vi "QPD Image Plane.vi"() -> ()   [LabVIEW 2018]
panel:
  in  "stop":bool
  out "Beam Centering 2":cluster{"Y":dbl[], "Y":dbl[]}[](graph) caption="Beam Centering"
  out "RF Offset A":dbl format="%0.6f"
  out "RF Offset C":dbl format="%0.6f"
  out "RF Offset B":dbl format="%0.6f"
  out "RF Offset D":dbl format="%0.6f"
  out "A":dynamicdata(graph)
  out "DC Offset A":dbl format="%0.6f"
  out "DC Offset C":dbl format="%0.6f"
  out "DC Offset B":dbl format="%0.6f"
  out "DC Offset D":dbl format="%0.6f"
  out "DC Responsivity D":dbl
  out "DC Responsivity C":dbl
  out "DC Responsivity B":dbl
  out "DC Responsivity A":dbl
  out "DC Responsivity D":dbl
  out "DC Responsivity C":dbl
  out "DC Responsivity B":dbl
  out "DC Responsivity A":dbl
  out "Y: (A+C)-(B+D)":dynamicdata(graph)
  out "X: (A+B)-(C+D)":dynamicdata(graph)
  out "D":dynamicdata(graph)
  out "B":dynamicdata(graph)
  out "C":dynamicdata(graph)
  out "Beam Centering":cluster{"Y":dbl[], "Y":dbl[]}[](graph)
  out "Y: (A+C)-(B+D)":dynamicdata(graph)
  out "X: (A+B)-(C+D)":dynamicdata(graph)
  out "Saving Data":bool
  out "Filename Out":path
  in  "Filename":path=path "C:/Users/physics-svc-fulda/Desktop/Data.lvm"
  in  "Enable":bool=TRUE
  out "D":dynamicdata(graph)
  out "B":dynamicdata(graph)
  out "C":dynamicdata(graph)
  out "A":dynamicdata(graph)
  in  "timeout (s)":dbl=10.0 format="%0.2f"
  in  "rate":dbl=1000.0
  in  "# of samples":i32=100
  out "Combined":dynamicdata(graph)
  # "Rayleigh Length"
  # "PZT Image Plane"
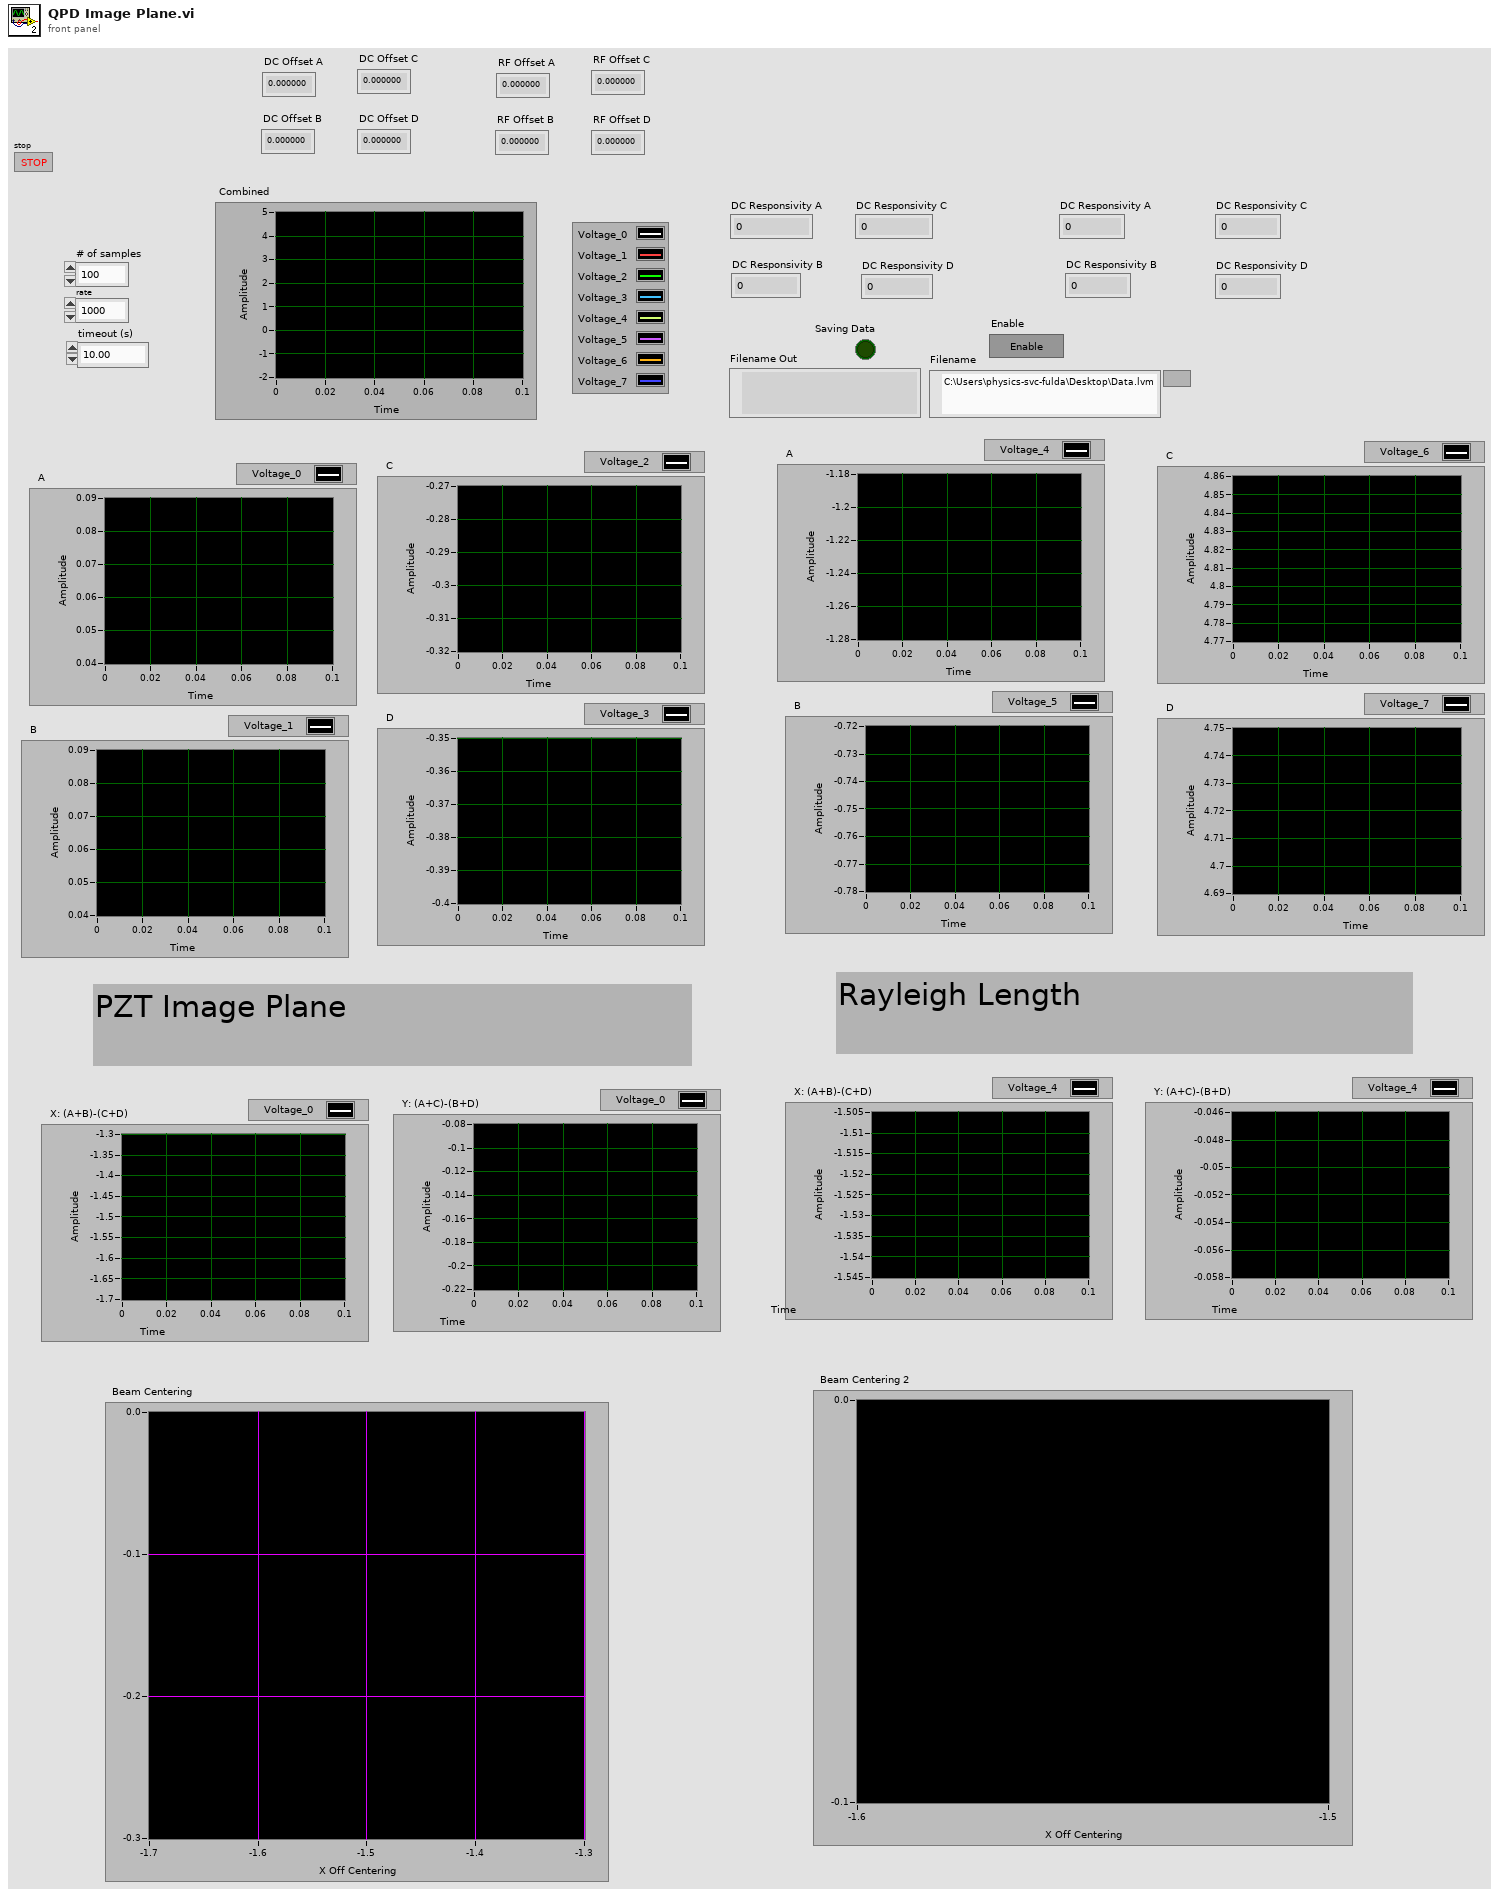
[diagram p1: front panel]
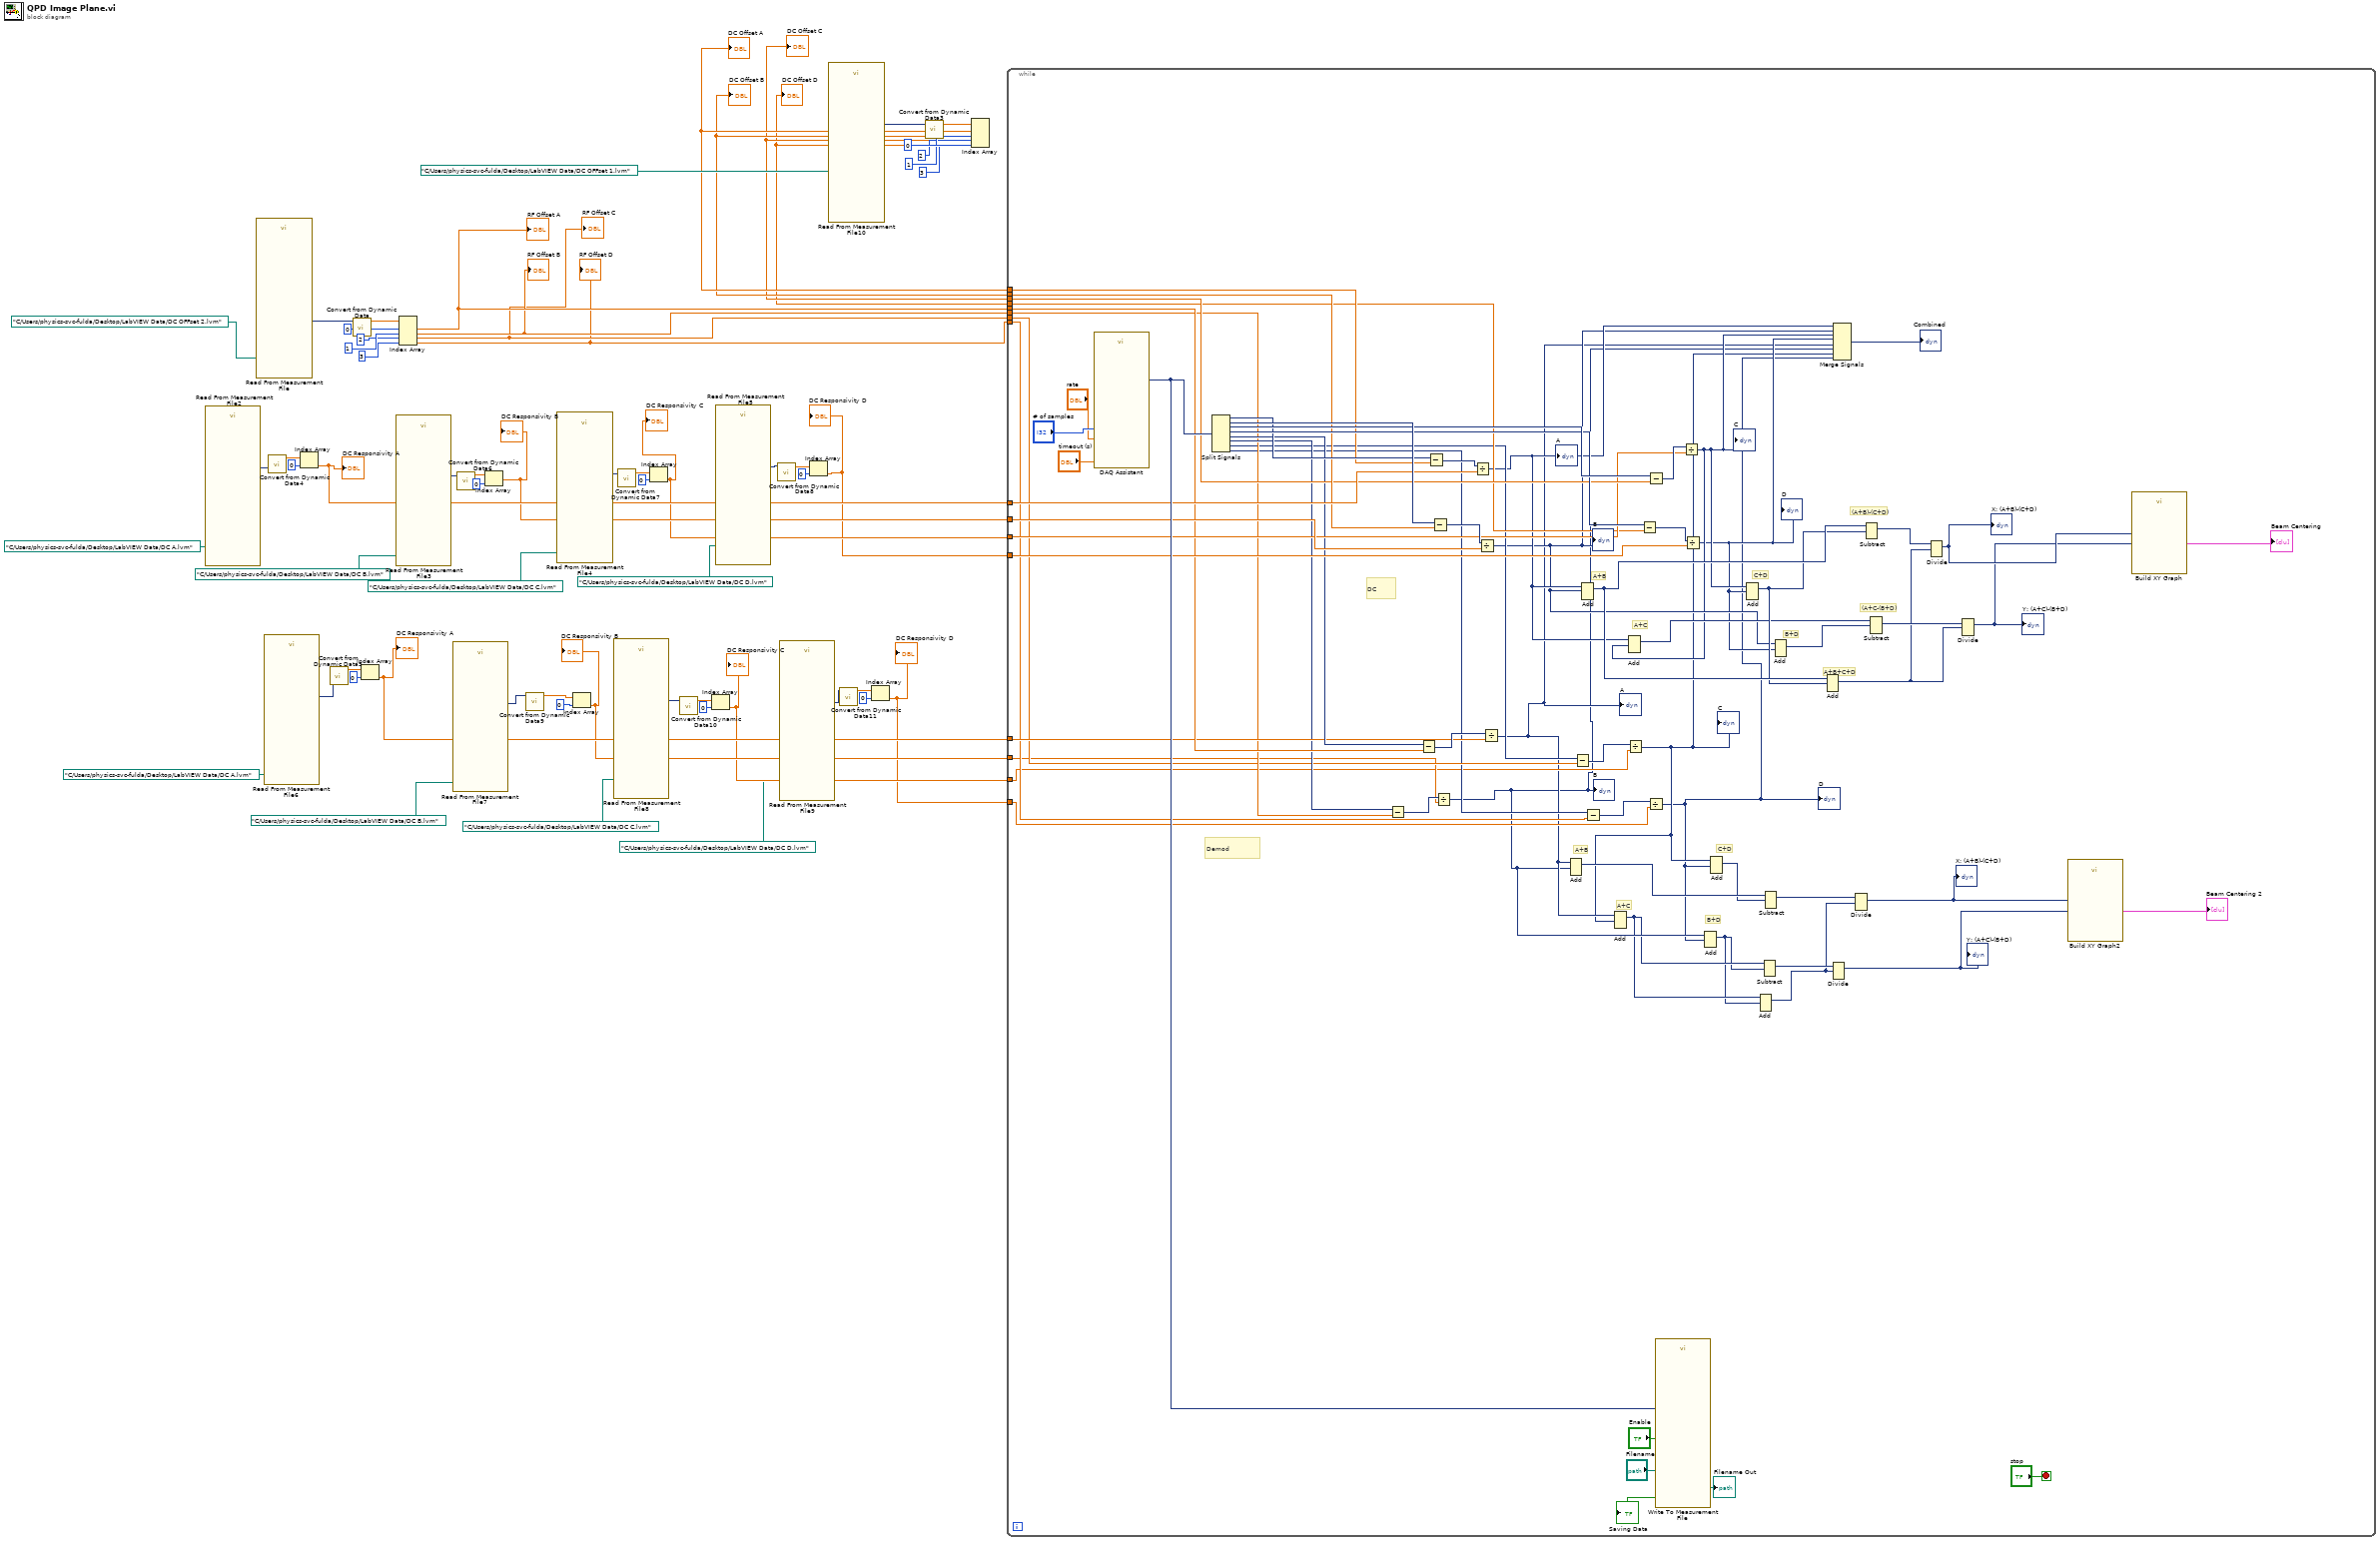
[diagram p0: block diagram]
diagram:
  n1 = call "Read From Measurement File2"("Filename"=path "C:/Users/physics-svc-fulda/Desktop/LabVIEW Data/DC A.lvm") -> ("Signals"=w46:dynamicdata)  [unwired: 5 in, 5 out]
  n2 = call "Read From Measurement File"("Filename"=path "C:/Users/physics-svc-fulda/Desktop/LabVIEW Data/DC OFFset 2.lvm") -> ("Signals"=w10:dynamicdata)  [unwired: 5 in, 5 out]
  n3 = call "Read From Measurement File6"("Filename"=path "C:/Users/physics-svc-fulda/Desktop/LabVIEW Data/DC A.lvm") -> ("Signals"=w49:dynamicdata)  [unwired: 5 in, 5 out]
  n4 = call "Convert from Dynamic Data4"("Dynamic Data Type"=w46) -> ("Array"=w47:dbl[])  [unwired: 3 in]
  n5 = Index Array(array=w47, index=0) -> (element=w31:dbl)
  "DC Responsivity A" <- w31
  n6 = call "Convert from Dynamic Data5"("Dynamic Data Type"=w49) -> ("Array"=w48:dbl[])  [unwired: 3 in]
  n7 = call "Convert from Dynamic Data"("Dynamic Data Type"=w10) -> ("Array"=w11:dbl[])  [unwired: 3 in]
  n8 = Index Array(array=w48, index=0) -> (element=w27:dbl)
  "DC Responsivity A" <- w27
  n9 = call "Read From Measurement File3"("Filename"=path "C:/Users/physics-svc-fulda/Desktop/LabVIEW Data/DC B.lvm") -> ("Signals"=w51:dynamicdata)  [unwired: 5 in, 5 out]
  n10 = Index Array(array=w11, index #1=0 ("index"), index #2=1 ("index"), index #3=2 ("index"), index #4=3 ("index")) -> (element #1=w4:dbl, element #2=w3:dbl, element #3=w2:dbl, element #4=w1:dbl)
  "RF Offset D" <- w1
  "RF Offset B" <- w3
  "RF Offset C" <- w2
  "RF Offset A" <- w4
  n11 = call "Read From Measurement File7"("Filename"=path "C:/Users/physics-svc-fulda/Desktop/LabVIEW Data/DC B.lvm") -> ("Signals"=w38:dynamicdata)  [unwired: 5 in, 5 out]
  n12 = call "Convert from Dynamic Data6"("Dynamic Data Type"=w51) -> ("Array"=w50:dbl[])  [unwired: 3 in]
  n13 = Index Array(array=w50, index=0) -> (element=w30:dbl)
  "DC Responsivity B" <- w30
  n14 = call "Convert from Dynamic Data9"("Dynamic Data Type"=w38) -> ("Array"=w40:dbl[])  [unwired: 3 in]
  n15 = call "Read From Measurement File4"("Filename"=path "C:/Users/physics-svc-fulda/Desktop/LabVIEW Data/DC C.lvm") -> ("Signals"=w53:dynamicdata)  [unwired: 5 in, 5 out]
  n16 = Index Array(array=w40, index=0) -> (element=w26:dbl)
  "DC Responsivity B" <- w26
  n17 = call "Read From Measurement File8"("Filename"=path "C:/Users/physics-svc-fulda/Desktop/LabVIEW Data/DC C.lvm") -> ("Signals"=w33:dynamicdata)  [unwired: 5 in, 5 out]
  n18 = call "Convert from Dynamic Data7"("Dynamic Data Type"=w53) -> ("Array"=w52:dbl[])  [unwired: 3 in]
  n19 = Index Array(array=w52, index=0) -> (element=w29:dbl)
  "DC Responsivity C" <- w29
  n20 = call "Convert from Dynamic Data10"("Dynamic Data Type"=w33) -> ("Array"=w37:dbl[])  [unwired: 3 in]
  n21 = Index Array(array=w37, index=0) -> (element=w25:dbl)
  "DC Responsivity C" <- w25
  n22 = call "Read From Measurement File5"("Filename"=path "C:/Users/physics-svc-fulda/Desktop/LabVIEW Data/DC D.lvm") -> ("Signals"=w55:dynamicdata)  [unwired: 5 in, 5 out]
  n23 = call "Convert from Dynamic Data8"("Dynamic Data Type"=w55) -> ("Array"=w54:dbl[])  [unwired: 3 in]
  n24 = call "Read From Measurement File9"("Filename"=path "C:/Users/physics-svc-fulda/Desktop/LabVIEW Data/DC D.lvm") -> ("Signals"=w32:dynamicdata)  [unwired: 5 in, 5 out]
  n25 = Index Array(array=w54, index=0) -> (element=w28:dbl)
  "DC Responsivity D" <- w28
  n26 = call "Read From Measurement File10"("Filename"=path "C:/Users/physics-svc-fulda/Desktop/LabVIEW Data/DC OFFset 1.lvm") -> ("Signals"=w61:dynamicdata)  [unwired: 5 in, 5 out]
  n27 = call "Convert from Dynamic Data11"("Dynamic Data Type"=w32) -> ("Array"=w35:dbl[])  [unwired: 3 in]
  n28 = Index Array(array=w35, index=0) -> (element=w24:dbl)
  "DC Responsivity D" <- w24
  n29 = call "Convert from Dynamic Data3"("Dynamic Data Type"=w61) -> ("Array"=w62:dbl[])  [unwired: 3 in]
  n30 = Index Array(array=w62, index #1=0 ("index"), index #2=1 ("index"), index #3=2 ("index"), index #4=3 ("index")) -> (element #1=w23:dbl, element #2=w22:dbl, element #3=w21:dbl, element #4=w20:dbl)
  "DC Offset D" <- w20
  "DC Offset B" <- w22
  "DC Offset C" <- w21
  "DC Offset A" <- w23
  n31 = while {
    tunnel: w23 -> [w106]
    tunnel: w22 -> [w104]
    tunnel: w21 -> [w102]
    tunnel: w20 -> [w100]
    tunnel: w4 -> [w97]
    tunnel: w3 -> [w92]
    tunnel: w2 -> [w89]
    tunnel: w1 -> [w86]
    tunnel: w31 -> [w105]
    tunnel: w30 -> [w103]
    tunnel: w29 -> [w101]
    tunnel: w28 -> [w99]
    tunnel: w27 -> [w95]
    tunnel: w26 -> [w85]
    tunnel: w25 -> [w84]
    tunnel: w24 -> [w83]
    stop <- "stop" stop-if-true
    # "B+D"
    # "A+C"
    # "C+D"
    # "A+B"
    # "(A+C-(B+D)"
    # "(A+B)-(C+D)"
    # "A+B+C+D"
    # "B+D"
    # "A+C"
    # "C+D"
    # "A+B"
    # "Demod"
    # "DC"
    n32 = call "DAQ Assistant"("rate"="rate", "number of samples"="# of samples", "timeout (s)"="timeout (s)") -> ("data"=w125:dynamicdata)  [unwired: 14 in, 2 out]
    n33 = Split Signals(w125) -> (w108:dynamicdata, w123:dynamicdata, w121:dynamicdata, w119:dynamicdata, w98:dynamicdata, w93:dynamicdata, w90:dynamicdata, w87:dynamicdata)  [unwired: 8 in]
    n34 = Subtract(x=w93, y=w92) -> (x-y=w94:dynamicdata)
    n35 = Subtract(x=w98, y=w97) -> (x-y=w96:dynamicdata)
    n36 = Subtract(x=w108, y=w106) -> (x-y=w107:dynamicdata)
    n37 = Subtract(x=w123, y=w104) -> (x-y=w122:dynamicdata)
    n38 = Divide(x=w94, y=w85) -> (x/y=w74:dynamicdata)
    "B" <- w74
    n39 = Divide(x=w107, y=w105) -> (x/y=w79:dynamicdata)
    "A" <- w79
    n40 = Divide(x=w122, y=w103) -> (x/y=w78:dynamicdata)
    "B" <- w78
    n41 = Divide(x=w96, y=w95) -> (x/y=w75:dynamicdata)
    "A" <- w75
    n42 = Add(1:w74, 2:w75) -> (0:w82:dynamicdata)  [unwired: 1 in, 1 out]
    n43 = Subtract(x=w90, y=w89) -> (x-y=w91:dynamicdata)
    n44 = Add(1:w78, 2:w79) -> (0:w117:dynamicdata)  [unwired: 1 in, 1 out]
    n45 = Subtract(x=w87, y=w86) -> (x-y=w88:dynamicdata)
    n46 = Divide(x=w91, y=w84) -> (x/y=w73:dynamicdata)
    "C" <- w73
    n47 = Add(1:w73, 2:w75) -> (0:w71:dynamicdata)  [unwired: 1 in, 1 out]
    n48 = Subtract(x=w119, y=w100) -> (x-y=w118:dynamicdata)
    n49 = Divide(x=w88, y=w83) -> (x/y=w72:dynamicdata)
    "D" <- w72
    n50 = Subtract(x=w121, y=w102) -> (x-y=w120:dynamicdata)
    n51 = call "Write To Measurement File"("Signals"=w125, "Enable"="Enable", "Filename"="Filename") -> ("Filename Out"=→"Filename Out":path, "Saving Data"=→"Saving Data":bool)  [unwired: 14 in, 1 out]
    n52 = Divide(x=w120, y=w101) -> (x/y=w77:dynamicdata)
    "C" <- w77
    n53 = Add(1:w77, 2:w79) -> (0:w114:dynamicdata)  [unwired: 1 in, 1 out]
    n54 = Divide(x=w118, y=w99) -> (x/y=w76:dynamicdata)
    "D" <- w76
    n55 = Add(1:w72, 2:w74) -> (0:w70:dynamicdata)  [unwired: 1 in, 1 out]
    n56 = Add(1:w72, 2:w73) -> (0:w81:dynamicdata)  [unwired: 1 in, 1 out]
    n57 = Add(1:w76, 2:w77) -> (0:w116:dynamicdata)  [unwired: 1 in, 1 out]
    n58 = Add(1:w70, 2:w71) -> (0:w67:dynamicdata)  [unwired: 1 in, 1 out]
    n59 = Subtract(1:w70, 2:w71) -> (0:w68:dynamicdata)  [unwired: 1 in, 1 out]
    n60 = Subtract(1:w81, 2:w82) -> (0:w69:dynamicdata)  [unwired: 1 in, 1 out]
    n61 = Add(1:w76, 2:w78) -> (0:w113:dynamicdata)  [unwired: 1 in, 1 out]
    n62 = Add(1:w116, 2:w117) -> (0:w111:dynamicdata)  [unwired: 1 in, 1 out]
    n63 = Divide(1:w67, 2:w68) -> (0:w64:dynamicdata)  [unwired: 1 in, 1 out]
    "Y: (A+C)-(B+D)" <- w64
    n64 = Merge Signals(w79, w78, w77, w76, w75, w74, w73, w72) -> (→"Combined":dynamicdata)
    n65 = Divide(1:w67, 2:w69) -> (0:w65:dynamicdata)  [unwired: 1 in, 1 out]
    "X: (A+B)-(C+D)" <- w65
    n66 = Subtract(1:w116, 2:w117) -> (0:w115:dynamicdata)  [unwired: 1 in, 1 out]
    n67 = Subtract(1:w113, 2:w114) -> (0:w112:dynamicdata)  [unwired: 1 in, 1 out]
    n68 = Divide(1:w111, 2:w115) -> (0:w110:dynamicdata)  [unwired: 1 in, 1 out]
    "X: (A+B)-(C+D)" <- w110
    n69 = Divide(1:w111, 2:w112) -> (0:w109:dynamicdata)  [unwired: 1 in, 1 out]
    "Y: (A+C)-(B+D)" <- w109
    n70 = call "Build XY Graph2"("Y Input"=w64, "X Input"=w65) -> ("XY Graph"=→"Beam Centering 2":cluster{"X":dbl[], "Y":dbl[]}[])  [unwired: 8 in, 1 out]
    n71 = call "Build XY Graph"("Y Input"=w109, "X Input"=w110) -> ("XY Graph"=→"Beam Centering":cluster{"X":dbl[], "Y":dbl[]}[])  [unwired: 8 in, 1 out]
  }
